vi "Burst Cell.vi"(0 "1D Board":T1[](array[typedef]), 5 "Team Number":i32, 7 "Index to Burst":i32, 11 "error in (no error)":errorcluster) -> (4 "1D Board Out":T1[](array[typedef]), 6 "Won?":bool, 8 "Coins Won":i32, 15 "error out":errorcluster)   [LabVIEW 2014, in "Dragon Tamers.lvlib"]
uses:
  Dragon Tamers.lvlib
  Typedefs/Board Cell.ctl
  Typedefs/Cell Occupancy.ctl
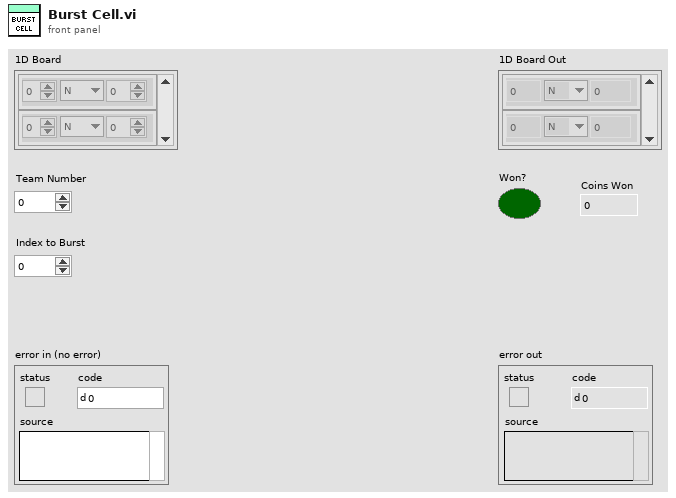
[diagram p1: front panel]
types:
  T1 = typedef "Dragon Tamers.lvlib/Board Cell.ctl" = cluster{"Team":i32, "Occu.":T2, "Count":i32}
  T2 = typedef "Dragon Tamers.lvlib/Cell Occupancy.ctl" = enum16{"N", "C", "K"}
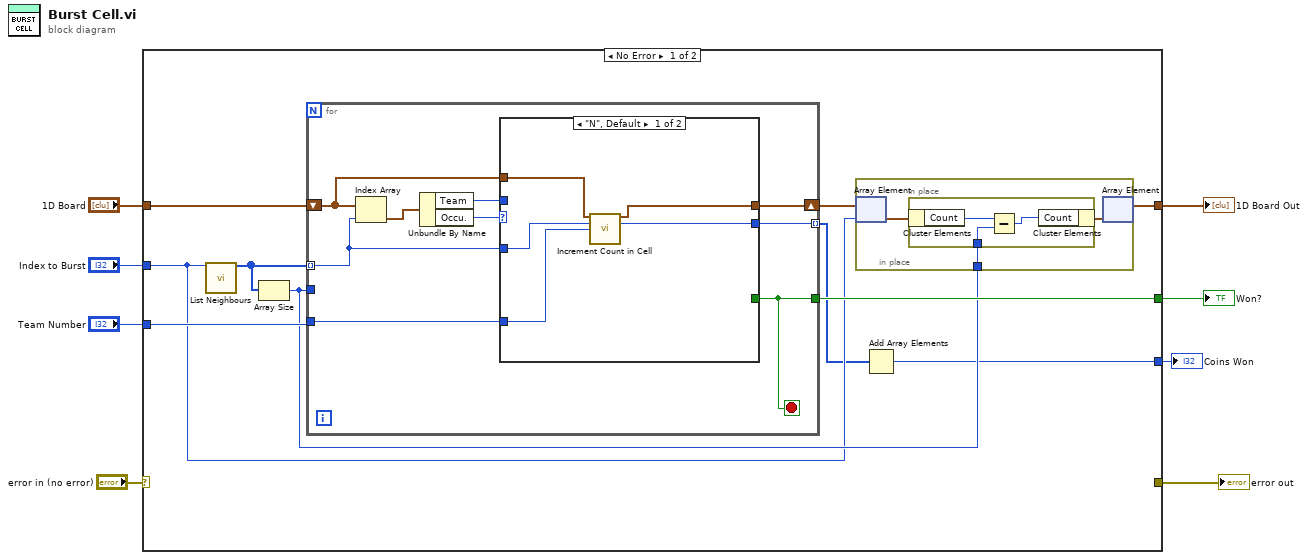
[diagram p0: block diagram]
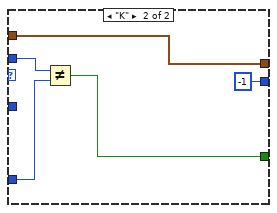
[diagram p2: hidden frame]
diagram:
  n1 = case shown="No Error" "error in (no error)" {
    selector: "error in (no error)" -> [_ w45]
    tunnel: [_ w45] -> w7
    tunnel: "1D Board" -> [w18 w44]
    tunnel: [w11 w44] -> w5
    tunnel: "Team Number" -> [w16 _]
    tunnel: "Index to Burst" -> [w13 _]
    tunnel: [w15 _] -> w2
    tunnel: [w9 _] -> w1
    frame No Error {
      n2 = call "List Neighbours.vi"("Cell Index"=w13) -> ("Neighbours"=w17:i32[])  [unwired: 12 in, 2 out]
      n3 = Array Size(array=w17) -> (size(s)=w14:i32)
      n4 = for {
        tunnel: w17 -> [w27] mode=indexing
        tunnel: w14 -> [_]
        tunnel: w16 -> [w30]
        tunnel: [w29] -> w15
        shift-right: [w26] -> w12
        shift-left: w18 -> [w28]
        tunnel: [w25] -> w10 mode=indexing
        stop <- w29 stop-if-true
        n5 = Index Array(array=w28, index=w27) -> (element=w33:T1)
        n6 = Unbundle By Name(w33) -> ("Team"=w31:i32, "Occu."=w32:T2)
        n7 = case shown="\"N\", Default" w32 {
          tunnel: w31 -> [_ w40]
          tunnel: w30 -> [w36 w41]
          tunnel: [_ w43] -> w29
          tunnel: w28 -> [w38 w42]
          tunnel: w27 -> [w37 _]
          tunnel: [w35 w42] -> w26
          tunnel: [w34 -1 ("Coins Won")] -> w25
          frame "N", Default {
            n8 = call "Increment Count in Cell.vi"("1D Board"=w38, "Cell Index"=w37, "Team Number"=w36) -> ("1D Board Out"=w35:T1[], "Coins Won"=w34:i32)  [unwired: 10 in, 1 out]
          }
          frame "K" {
            n9 = Not Equal?(x=w40, y=w41) -> (x != y?=w43:bool)
          }
        }
      }
      n10 = in-place {
        in-place-border: w14 -> [w21]
        n11 = in-place-array #1(w12, w13) -> (w20:T1)
        n12 = in-place {
          in-place-border: w21 -> [w23]
          n13 = in-place-cluster #2(w20) -> ("Count"=w24:i32)
          n14 = Subtract(x=w24, y=w23) -> (x-y=w22:i32)
          n15 = in-place-cluster #2("Count"=w22) -> (w19:T1)
        }
        n16 = in-place-array #1(w19) -> (w11:T1[])  [unwired: 1 out]
      }
      n17 = Add Array Elements(numeric array=w10) -> (sum=w9:i32)
    }
    frame Error {
    }
  }
  "error out" <- w7
  "1D Board Out" <- w5
  "Won?" <- w2
  "Coins Won" <- w1
